vi "Get Block Data Ref.vi"(8 "error in (no error)":errorcluster, 11 "Simulated VeriStand Engine in":refnum<class "Simulated VeriStand Engine.lvclass">) -> (0 "error out":errorcluster, 2 "Block Data Ref":T1[](array[typedef]) {"Data Reference" format="%.0x"}, 3 "Simulated VeriStand Engine out":refnum<class "Simulated VeriStand Engine.lvclass">)   [LabVIEW 2016, in "Simulated VeriStand Engine.lvclass"]
uses:
  Simulated VeriStand Engine.lvclass
  <vilib>/NI Veristand/Custom Device API/Block Data Reference.ctl
  <vilib>/NI Veristand/Custom Device API/Data Reference.ctl
  Simulated VeriStand Engine.lvclass/Simulated VeriStand Engine.ctl
  <vilib>/NI Veristand/Custom Device API/Custom Device API.lvlib
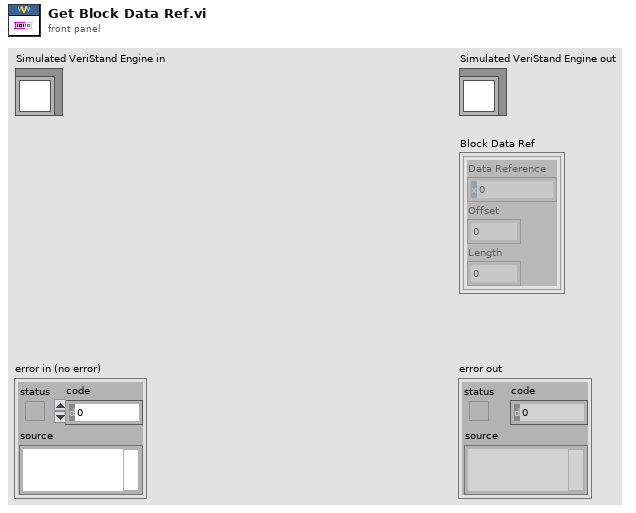
[diagram p1: front panel]
types:
  T1 = typedef "Custom Device API.lvlib/Block Data Reference.ctl" = cluster{"Data Reference":T2, "Offset":u64, "Length":u64}
  T2 = typedef "Custom Device API.lvlib/Data Reference.ctl" = i32
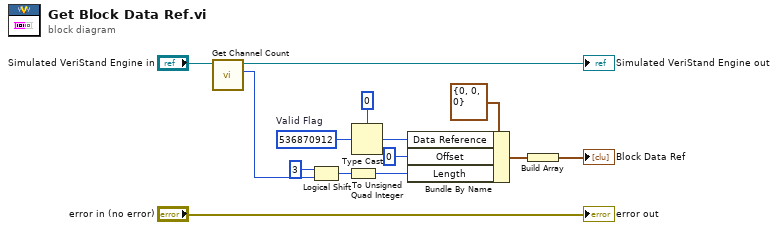
[diagram p0: block diagram]
diagram:
  w12 = 536870912  # Valid Flag
  n1 = call "Get Channel Count.vi"("Simulated VeriStand Engine in"="Simulated VeriStand Engine in") -> ("Channel Count"=w5:u32, "Simulated VeriStand Engine out"=→"Simulated VeriStand Engine out":refnum<class "Simulated VeriStand Engine.lvclass">)  [unwired: 8 in, 1 out]
  n2 = Logical Shift(y=i16 3, x=w5) -> (x << y=w3:u32)
  n3 = To Unsigned Quad Integer(1:w3) -> (0:w2:u64)
  n4 = Type Cast(type=T2 0 ("Data Reference"), x=w12) -> (*(type *) &x=w14:T2)
  n5 = Bundle By Name(cluster=T1 {"Data Reference"=0, "Offset"=0, "Length"=0} ("Block Data Ref"), "Data Reference"=w14, "Offset"=u64 0, "Length"=w2) -> (w11:T1)
  n6 = Build Array(w11) -> (→"Block Data Ref":T1[])
  "error out" <- "error in (no error)"
